vi "FdxCmdRxUDPBlockReadCvi.vi"(8 "error in":errorcluster, 9 "RxUDPBlockReadInPortArray":T1[](array[typedef]) {"UDP Handle Out" format="%.0x"; "UDP Handle" format="%.0x"}, 10 "PortCountIn":u32, 11 "InstrumentHandle_port":u32=4) -> (0 "error out":errorcluster, 1 "RxUDPBlockReadInPortArray":T1[](array[typedef]) {"UDP Handle Out" format="%.0x"; "UDP Handle" format="%.0x"}, 3 "InstrumentHandle_port":u32)   [LabVIEW 2020, in "AIM664LV.lvlib"]
doc: "This function reads data from one or several UDP connection oriented ports."
uses:
  AIM664LV.lvlib
  AFDX_Controls/ReceiveUDPBlockRead.ctl
  AFDX_LibraryAdmin/FdxGlobalDllPath.vi
panel:
  out "UdpBlockReadOut":T2
  in  "UdpBlockReadIn":T3={"PortCountIn"=4, "UdpBlockReadInPortArray"=[548424, 1, 583608, 1, 584000, 1, 584144, 1]}
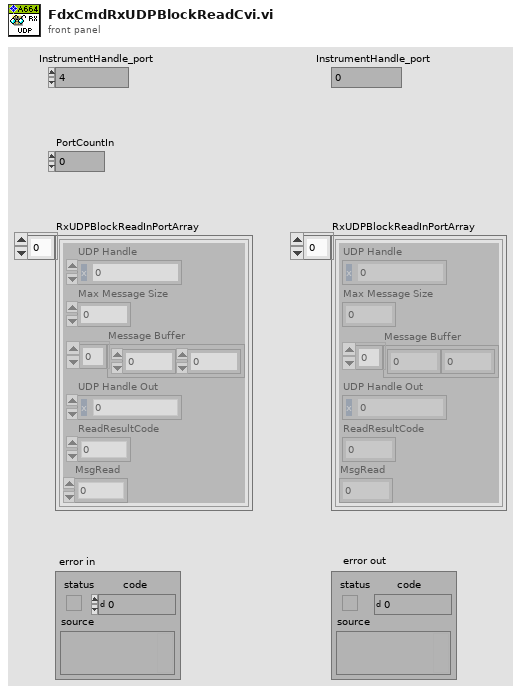
[diagram p1: front panel]
types:
  T1 = typedef "AIM664LV.lvlib/ReceiveUDPBlockRead.ctl" = cluster{"UDP Handle":u32, "Max Message Size":u32, "Message Buffer":u8[], "UDP Handle Out":u32, "ReadResultCode":i32, "MsgRead":u32}
  T2 = cluster{"PortCountOut":u32, "UdpBlockReadOutPortArray":u32[]}
  T3 = cluster{"PortCountIn":u32, "UdpBlockReadInPortArray":u32[]}
  T4 = cluster{"RxUDPBlockReadInPortArray[0]":T1, "RxUDPBlockReadInPortArray[1]":T1, "RxUDPBlockReadInPortArray[2]":T1, "RxUDPBlockReadInPortArray[3]":T1, "RxUDPBlockReadInPortArray[4]":T1, "RxUDPBlockReadInPortArray[5]":T1, "RxUDPBlockReadInPortArray[6]":T1, "RxUDPBlockReadInPortArray[7]":T1, "RxUDPBlockReadInPortArray[8]":T1, "RxUDPBlockReadInPortArray[9]":T1, "RxUDPBlockReadInPortArray[10]":T1, "RxUDPBlockReadInPortArray[11]":T1, "RxUDPBlockReadInPortArray[12]":T1, "RxUDPBlockReadInPortArray[13]":T1, "RxUDPBlockReadInPortArray[14]":T1, "RxUDPBlockReadInPortArray[15]":T1, "RxUDPBlockReadInPortArray[16]":T1, "RxUDPBlockReadInPortArray[17]":T1, "RxUDPBlockReadInPortArray[18]":T1, "RxUDPBlockReadInPortArray[19]":T1, "RxUDPBlockReadInPortArray[20]":T1, "RxUDPBlockReadInPortArray[21]":T1, "RxUDPBlockReadInPortArray[22]":T1, "RxUDPBlockReadInPortArray[23]":T1, "RxUDPBlockReadInPortArray[24]":T1, "RxUDPBlockReadInPortArray[25]":T1, "RxUDPBlockReadInPortArray[26]":T1, "RxUDPBlockReadInPortArray[27]":T1, "RxUDPBlockReadInPortArray[28]":T1, "RxUDPBlockReadInPortArray[29]":T1, "RxUDPBlockReadInPortArray[30]":T1, "RxUDPBlockReadInPortArray[31]":T1, "RxUDPBlockReadInPortArray[32]":T1, "RxUDPBlockReadInPortArray[33]":T1, "RxUDPBlockReadInPortArray[34]":T1, "RxUDPBlockReadInPortArray[35]":T1, "RxUDPBlockReadInPortArray[36]":T1, "RxUDPBlockReadInPortArray[37]":T1, "RxUDPBlockReadInPortArray[38]":T1, "RxUDPBlockReadInPortArray[39]":T1, "RxUDPBlockReadInPortArray[40]":T1, "RxUDPBlockReadInPortArray[41]":T1, "RxUDPBlockReadInPortArray[42]":T1, "RxUDPBlockReadInPortArray[43]":T1, "RxUDPBlockReadInPortArray[44]":T1, "RxUDPBlockReadInPortArray[45]":T1, "RxUDPBlockReadInPortArray[46]":T1, "RxUDPBlockReadInPortArray[47]":T1, "RxUDPBlockReadInPortArray[48]":T1, "RxUDPBlockReadInPortArray[49]":T1, "RxUDPBlockReadInPortArray[50]":T1, "RxUDPBlockReadInPortArray[51]":T1, "RxUDPBlockReadInPortArray[52]":T1, "RxUDPBlockReadInPortArray[53]":T1, "RxUDPBlockReadInPortArray[54]":T1, "RxUDPBlockReadInPortArray[55]":T1, "RxUDPBlockReadInPortArray[56]":T1, "RxUDPBlockReadInPortArray[57]":T1, "RxUDPBlockReadInPortArray[58]":T1, "RxUDPBlockReadInPortArray[59]":T1, "RxUDPBlockReadInPortArray[60]":T1, "RxUDPBlockReadInPortArray[61]":T1, "RxUDPBlockReadInPortArray[62]":T1, "RxUDPBlockReadInPortArray[63]":T1, "RxUDPBlockReadInPortArray[64]":T1, "RxUDPBlockReadInPortArray[65]":T1, "RxUDPBlockReadInPortArray[66]":T1, "RxUDPBlockReadInPortArray[67]":T1, "RxUDPBlockReadInPortArray[68]":T1, "RxUDPBlockReadInPortArray[69]":T1, "RxUDPBlockReadInPortArray[70]":T1, "RxUDPBlockReadInPortArray[71]":T1, "RxUDPBlockReadInPortArray[72]":T1, "RxUDPBlockReadInPortArray[73]":T1, "RxUDPBlockReadInPortArray[74]":T1, "RxUDPBlockReadInPortArray[75]":T1, "RxUDPBlockReadInPortArray[76]":T1, "RxUDPBlockReadInPortArray[77]":T1, "RxUDPBlockReadInPortArray[78]":T1, "RxUDPBlockReadInPortArray[79]":T1, "RxUDPBlockReadInPortArray[80]":T1, "RxUDPBlockReadInPortArray[81]":T1, "RxUDPBlockReadInPortArray[82]":T1, "RxUDPBlockReadInPortArray[83]":T1, "RxUDPBlockReadInPortArray[84]":T1, "RxUDPBlockReadInPortArray[85]":T1, "RxUDPBlockReadInPortArray[86]":T1, "RxUDPBlockReadInPortArray[87]":T1, "RxUDPBlockReadInPortArray[88]":T1, "RxUDPBlockReadInPortArray[89]":T1, "RxUDPBlockReadInPortArray[90]":T1, "RxUDPBlockReadInPortArray[91]":T1, "RxUDPBlockReadInPortArray[92]":T1, "RxUDPBlockReadInPortArray[93]":T1, "RxUDPBlockReadInPortArray[94]":T1, "RxUDPBlockReadInPortArray[95]":T1, "RxUDPBlockReadInPortArray[96]":T1, "RxUDPBlockReadInPortArray[97]":T1, "RxUDPBlockReadInPortArray[98]":T1, "RxUDPBlockReadInPortArray[99]":T1, "RxUDPBlockReadInPortArray[100]":T1, "RxUDPBlockReadInPortArray[101]":T1, "RxUDPBlockReadInPortArray[102]":T1, "RxUDPBlockReadInPortArray[103]":T1, "RxUDPBlockReadInPortArray[104]":T1, "RxUDPBlockReadInPortArray[105]":T1, "RxUDPBlockReadInPortArray[106]":T1, "RxUDPBlockReadInPortArray[107]":T1, "RxUDPBlockReadInPortArray[108]":T1, "RxUDPBlockReadInPortArray[109]":T1, "RxUDPBlockReadInPortArray[110]":T1, "RxUDPBlockReadInPortArray[111]":T1, "RxUDPBlockReadInPortArray[112]":T1, "RxUDPBlockReadInPortArray[113]":T1, "RxUDPBlockReadInPortArray[114]":T1, "RxUDPBlockReadInPortArray[115]":T1, "RxUDPBlockReadInPortArray[116]":T1, "RxUDPBlockReadInPortArray[117]":T1, "RxUDPBlockReadInPortArray[118]":T1, "RxUDPBlockReadInPortArray[119]":T1, "RxUDPBlockReadInPortArray[120]":T1, "RxUDPBlockReadInPortArray[121]":T1, "RxUDPBlockReadInPortArray[122]":T1, "RxUDPBlockReadInPortArray[123]":T1, "RxUDPBlockReadInPortArray[124]":T1, "RxUDPBlockReadInPortArray[125]":T1, "RxUDPBlockReadInPortArray[126]":T1, "RxUDPBlockReadInPortArray[127]":T1, "RxUDPBlockReadInPortArray[128]":T1, "RxUDPBlockReadInPortArray[129]":T1, "RxUDPBlockReadInPortArray[130]":T1, "RxUDPBlockReadInPortArray[131]":T1, "RxUDPBlockReadInPortArray[132]":T1, "RxUDPBlockReadInPortArray[133]":T1, "RxUDPBlockReadInPortArray[134]":T1, "RxUDPBlockReadInPortArray[135]":T1, "RxUDPBlockReadInPortArray[136]":T1, "RxUDPBlockReadInPortArray[137]":T1, "RxUDPBlockReadInPortArray[138]":T1, "RxUDPBlockReadInPortArray[139]":T1, "RxUDPBlockReadInPortArray[140]":T1, "RxUDPBlockReadInPortArray[141]":T1, "RxUDPBlockReadInPortArray[142]":T1, "RxUDPBlockReadInPortArray[143]":T1, "RxUDPBlockReadInPortArray[144]":T1, "RxUDPBlockReadInPortArray[145]":T1, "RxUDPBlockReadInPortArray[146]":T1, "RxUDPBlockReadInPortArray[147]":T1, "RxUDPBlockReadInPortArray[148]":T1, "RxUDPBlockReadInPortArray[149]":T1, "RxUDPBlockReadInPortArray[150]":T1, "RxUDPBlockReadInPortArray[151]":T1, "RxUDPBlockReadInPortArray[152]":T1, "RxUDPBlockReadInPortArray[153]":T1, "RxUDPBlockReadInPortArray[154]":T1, "RxUDPBlockReadInPortArray[155]":T1, "RxUDPBlockReadInPortArray[156]":T1, "RxUDPBlockReadInPortArray[157]":T1, "RxUDPBlockReadInPortArray[158]":T1, "RxUDPBlockReadInPortArray[159]":T1, "RxUDPBlockReadInPortArray[160]":T1, "RxUDPBlockReadInPortArray[161]":T1, "RxUDPBlockReadInPortArray[162]":T1, "RxUDPBlockReadInPortArray[163]":T1, "RxUDPBlockReadInPortArray[164]":T1, "RxUDPBlockReadInPortArray[165]":T1, "RxUDPBlockReadInPortArray[166]":T1, "RxUDPBlockReadInPortArray[167]":T1, "RxUDPBlockReadInPortArray[168]":T1, "RxUDPBlockReadInPortArray[169]":T1, "RxUDPBlockReadInPortArray[170]":T1, "RxUDPBlockReadInPortArray[171]":T1, "RxUDPBlockReadInPortArray[172]":T1, "RxUDPBlockReadInPortArray[173]":T1, "RxUDPBlockReadInPortArray[174]":T1, "RxUDPBlockReadInPortArray[175]":T1, "RxUDPBlockReadInPortArray[176]":T1, "RxUDPBlockReadInPortArray[177]":T1, "RxUDPBlockReadInPortArray[178]":T1, "RxUDPBlockReadInPortArray[179]":T1, "RxUDPBlockReadInPortArray[180]":T1, "RxUDPBlockReadInPortArray[181]":T1, "RxUDPBlockReadInPortArray[182]":T1, "RxUDPBlockReadInPortArray[183]":T1, "RxUDPBlockReadInPortArray[184]":T1, "RxUDPBlockReadInPortArray[185]":T1, "RxUDPBlockReadInPortArray[186]":T1, "RxUDPBlockReadInPortArray[187]":T1, "RxUDPBlockReadInPortArray[188]":T1, "RxUDPBlockReadInPortArray[189]":T1, "RxUDPBlockReadInPortArray[190]":T1, "RxUDPBlockReadInPortArray[191]":T1, "RxUDPBlockReadInPortArray[192]":T1, "RxUDPBlockReadInPortArray[193]":T1, "RxUDPBlockReadInPortArray[194]":T1, "RxUDPBlockReadInPortArray[195]":T1, "RxUDPBlockReadInPortArray[196]":T1, "RxUDPBlockReadInPortArray[197]":T1, "RxUDPBlockReadInPortArray[198]":T1, "RxUDPBlockReadInPortArray[199]":T1, "RxUDPBlockReadInPortArray[200]":T1, "RxUDPBlockReadInPortArray[201]":T1, "RxUDPBlockReadInPortArray[202]":T1, "RxUDPBlockReadInPortArray[203]":T1, "RxUDPBlockReadInPortArray[204]":T1, "RxUDPBlockReadInPortArray[205]":T1, "RxUDPBlockReadInPortArray[206]":T1, "RxUDPBlockReadInPortArray[207]":T1, "RxUDPBlockReadInPortArray[208]":T1, "RxUDPBlockReadInPortArray[209]":T1, "RxUDPBlockReadInPortArray[210]":T1, "RxUDPBlockReadInPortArray[211]":T1, "RxUDPBlockReadInPortArray[212]":T1, "RxUDPBlockReadInPortArray[213]":T1, "RxUDPBlockReadInPortArray[214]":T1, "RxUDPBlockReadInPortArray[215]":T1, "RxUDPBlockReadInPortArray[216]":T1, "RxUDPBlockReadInPortArray[217]":T1, "RxUDPBlockReadInPortArray[218]":T1, "RxUDPBlockReadInPortArray[219]":T1, "RxUDPBlockReadInPortArray[220]":T1, "RxUDPBlockReadInPortArray[221]":T1, "RxUDPBlockReadInPortArray[222]":T1, "RxUDPBlockReadInPortArray[223]":T1, "RxUDPBlockReadInPortArray[224]":T1, "RxUDPBlockReadInPortArray[225]":T1, "RxUDPBlockReadInPortArray[226]":T1, "RxUDPBlockReadInPortArray[227]":T1, "RxUDPBlockReadInPortArray[228]":T1, "RxUDPBlockReadInPortArray[229]":T1, "RxUDPBlockReadInPortArray[230]":T1, "RxUDPBlockReadInPortArray[231]":T1, "RxUDPBlockReadInPortArray[232]":T1, "RxUDPBlockReadInPortArray[233]":T1, "RxUDPBlockReadInPortArray[234]":T1, "RxUDPBlockReadInPortArray[235]":T1, "RxUDPBlockReadInPortArray[236]":T1, "RxUDPBlockReadInPortArray[237]":T1, "RxUDPBlockReadInPortArray[238]":T1, "RxUDPBlockReadInPortArray[239]":T1, "RxUDPBlockReadInPortArray[240]":T1, "RxUDPBlockReadInPortArray[241]":T1, "RxUDPBlockReadInPortArray[242]":T1, "RxUDPBlockReadInPortArray[243]":T1, "RxUDPBlockReadInPortArray[244]":T1, "RxUDPBlockReadInPortArray[245]":T1, "RxUDPBlockReadInPortArray[246]":T1, "RxUDPBlockReadInPortArray[247]":T1, "RxUDPBlockReadInPortArray[248]":T1, "RxUDPBlockReadInPortArray[249]":T1, "RxUDPBlockReadInPortArray[250]":T1, "RxUDPBlockReadInPortArray[251]":T1, "RxUDPBlockReadInPortArray[252]":T1, "RxUDPBlockReadInPortArray[253]":T1, "RxUDPBlockReadInPortArray[254]":T1, "RxUDPBlockReadInPortArray[255]":T1}
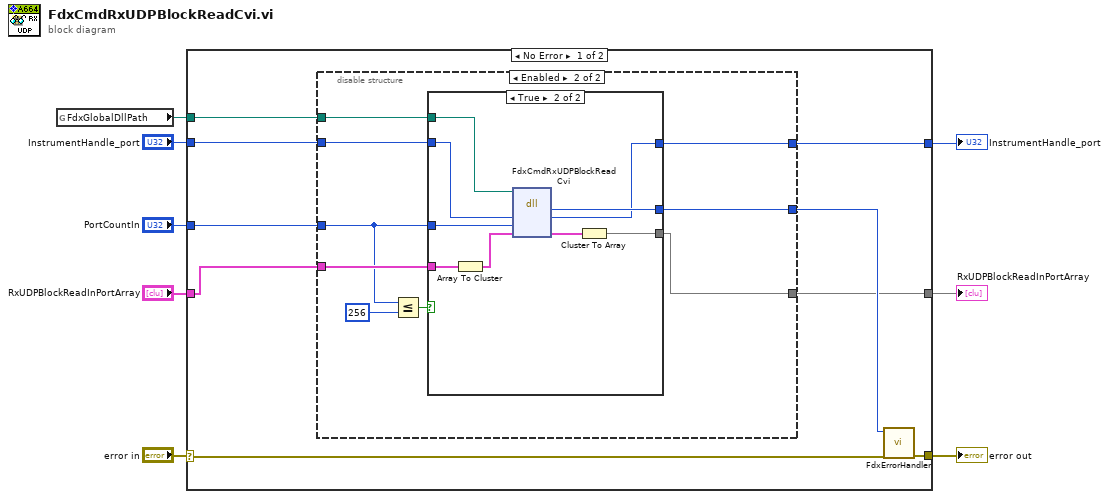
[diagram p0: block diagram]
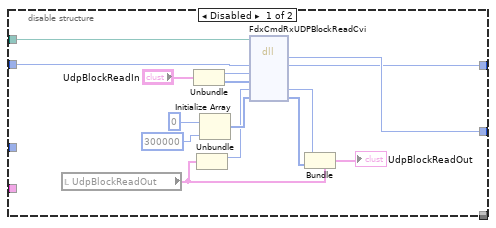
[diagram p2: hidden frame]
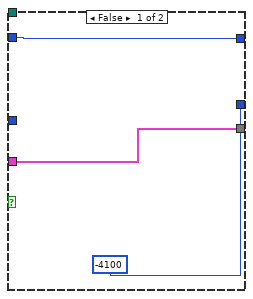
[diagram p3: hidden frame]
diagram:
  n1 = global read "FdxGlobalDllPath.vi" "FdxGlobalDllPath"() -> (w6:path)
  n2 = case shown="No Error" "error in" {
    selector: "error in" -> [w16 w56]
    tunnel: [w17 w56] -> w8
    tunnel: w6 -> [w14 _]
    tunnel: "InstrumentHandle_port" -> [w13 w55]
    tunnel: [w12 w55] -> w4
    tunnel: "RxUDPBlockReadInPortArray" -> [w11 w54]
    tunnel: "PortCountIn" -> [w10 _]
    tunnel: [w9 w54] -> w1
    frame No Error {
      n3 = disable-structure shown="Enabled" {
        disable-tunnel: [w32 w37] -> w15
        disable-tunnel: w14 -> [w20 w39]
        disable-tunnel: w13 -> [w19 w38]
        disable-tunnel: [w18 w33] -> w12
        disable-tunnel: w11 -> [_ w36]
        disable-tunnel: w10 -> [_ w35]
        disable-tunnel: [_ w34] -> w9
        frame Disabled {
          n4 = local read "UdpBlockReadOut"() -> (w21:T2)
          n5 = Unbundle("UdpBlockReadIn") -> ("PortCountIn"=w30:u32, "UdpBlockReadInPortArray"=w27:u32[])
          n6 = Unbundle(w21) -> ("PortCountOut"=w22:u32)  [unwired: 1 out]
          n7 = Initialize Array(u32 0 ("element"), 300000 ("dimension size")) -> (w23:u32[])
          n8 = dll-call lib="aim_fdx.19.dll" fn="FdxCmdRxUDPBlockReadCvi"(path in=w20, "InstrumentHandle"=w19, "PortCountIn"=w30, "UdpBlockReadInPortArray"=w27, "PortCountOut"=w22, "UdpBlockReadOutPortArray"=w23) -> ("status"=w32:i32, "InstrumentHandle"=w18:u32, "PortCountOut"=w29:u32, "UdpBlockReadOutPortArray"=w28:u32[])  [unwired: 4 in, 2 out]
          n9 = Bundle(cluster=w21, "PortCountOut"=w29, "UdpBlockReadOutPortArray"=w28) -> (→"UdpBlockReadOut":T2)
        }
        frame Enabled {
          n10 = Less Or Equal?(x=w35, y=u32 256) -> (x <= y?=w40:bool)
          n11 = case shown="True" w40 {
            tunnel: [-4100 ("status") w53] -> w37
            tunnel: w38 -> [w42 w52]
            tunnel: w39 -> [_ w51]
            tunnel: [w44 w49] -> w34
            tunnel: w35 -> [_ w48]
            tunnel: w36 -> [w44 w47]
            tunnel: [w42 w45] -> w33
            frame False {
            }
            frame True {
              n12 = Array To Cluster(array=w47) -> (cluster=w46:T4)
              n13 = dll-call lib="aim_fdx.19.dll" fn="FdxCmdRxUDPBlockReadCvi"(path in=w51, "InstrumentHandle"=w52, "PortCountIn"=w48, "UdpBlockReadInPortArray"=w46) -> ("status"=w53:i32, "InstrumentHandle"=w45:u32, "UdpBlockReadInPortArray"=w50:T4)  [unwired: 3 in, 2 out]
              n14 = Cluster To Array(cluster=w50) -> (array=w49:T1[])
            }
          }
        }
      }
      n15 = call "FdxErrorHandler.vi"("error in"=w16, "AIM Error"=w15) -> ("error out"=w17:errorcluster)  [unwired: 9 in]
    }
    frame Error {
    }
  }
  "error out" <- w8
  "InstrumentHandle_port" <- w4
  "RxUDPBlockReadInPortArray" <- w1
